vi "look arond me.vi"(9 "Position":T1, 10 "map":T2[][](array[typedef])) -> (2 "index_out":cluster{"Numeric":i32, "Numeric":i32}[](array[cluster]), 3 "map data of it":T2[](array[typedef]))   [LabVIEW 2020, in "The_Hill_Youth.lvlib" / "MySquare.lvclass"]
uses:
  MySquare.lvclass
  MyTeam/map_point.ctl
  SquareBattle/Position.ctl
  SquareBattle/SquareBattle.lvlib
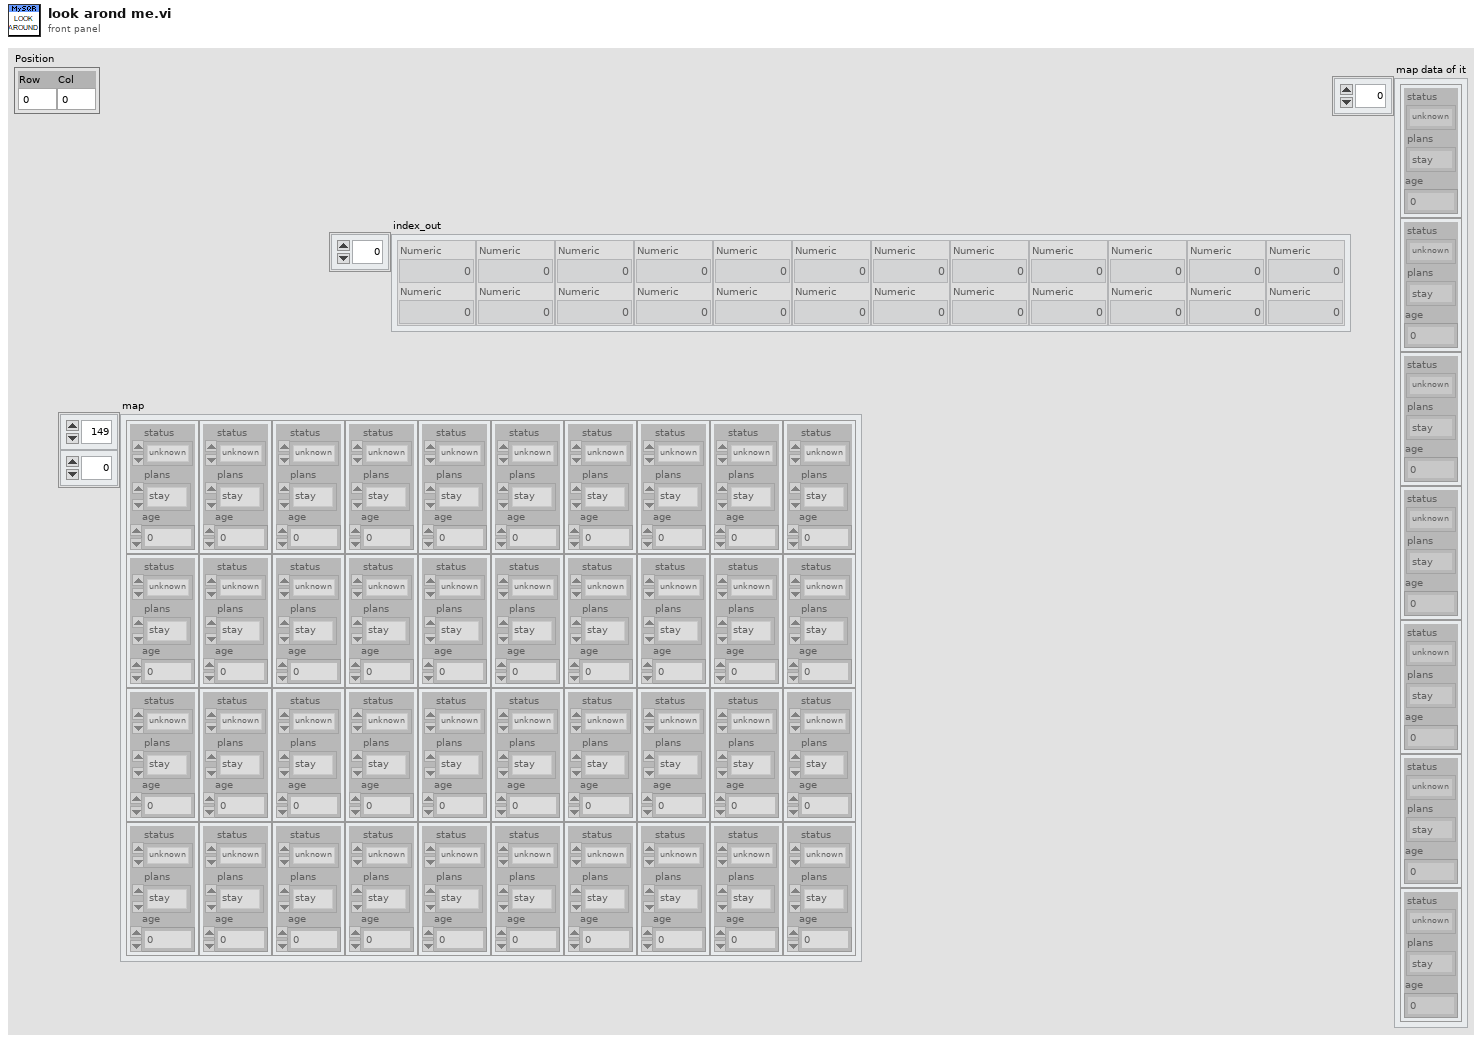
[diagram p1: front panel]
types:
  T1 = typedef "SquareBattle.lvlib/Position.ctl" = cluster{"Row":i32, "Col":i32}
  T2 = typedef "map_point.ctl" = cluster{"status":enum16{"unknown", "frind", "enemy", "empty"}, "plans":enum16{"stay", "duplicate", "attack", "move to", "no plans"}, "age":dbl}
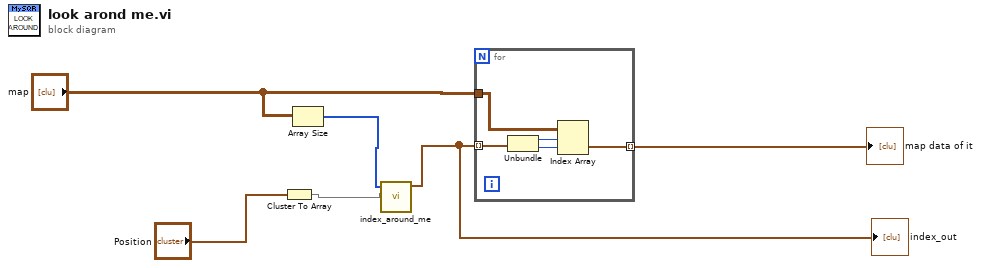
[diagram p0: block diagram]
diagram:
  n1 = Cluster To Array(cluster="Position") -> (array=w6:i32[])
  n2 = Array Size(array="map") -> (size(s)=w5:i32[])
  n3 = call "index_around_me.vi"("my position"=w6, "board_size"=w5) -> ("index_out"=w4:cluster{"Numeric":i32, "Numeric":i32}[])  [unwired: 9 in]
  "index_out" <- w4
  n4 = for {
    tunnel: w4 -> [w11] mode=indexing
    tunnel: "map" -> [w10]
    tunnel: [w7] -> w2 mode=indexing
    n5 = Unbundle(w11) -> ("Numeric"=w9:i32, "Numeric"=w8:i32)
    n6 = Index Array(array=w10, index (row)=w9, index (col)=w8) -> (element=w7:T2)
  }
  "map data of it" <- w2
